vi "File Read Binary File.vi"(5 "count":i32=-1, 6 "字节顺序":T1(ring)=enum."little-endian", 8 "error in":errorcluster, 9 "access":enum16{"read/write", "read-only", "write-only"}(ring)=enum."read-only", 10 "operation":T2(ring), 11 "file path":path) -> (0 "error Output":errorcluster, 2 "Variant Output":variant, 3 "path":path)   [LabVIEW 2018]
doc: "从字节流二进制文件中读取数据数组。默认情况下，VI被配置为读取8字节Little Endian数据（双精度长整型DBL）。要修改从文件中读取采样数据的方式，可修改字节顺序和字节大小的值（通常大小为1、2、4或8）。如修改字节大小，也需修改数据类型常量的表示法，使其与字节大小相一致（1 = I8、2 = I16、4 = I32、8 = DBL）。用“写入二进制文件”VI创建文件。"
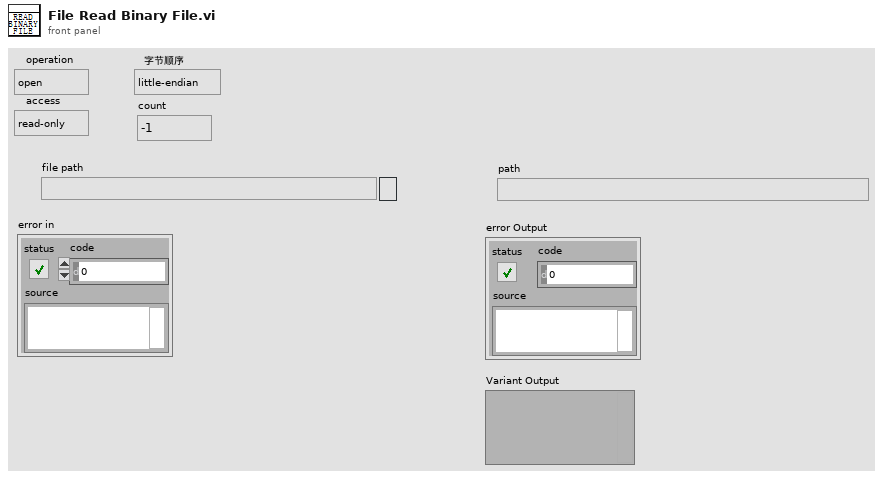
[diagram p1: front panel]
types:
  T1 = enum16{"big-endian, network order", "native, host order", "little-endian"}
  T2 = enum16{"open", "replace", "create", "open or create", "replace or create", "replace or create with confirmation"}
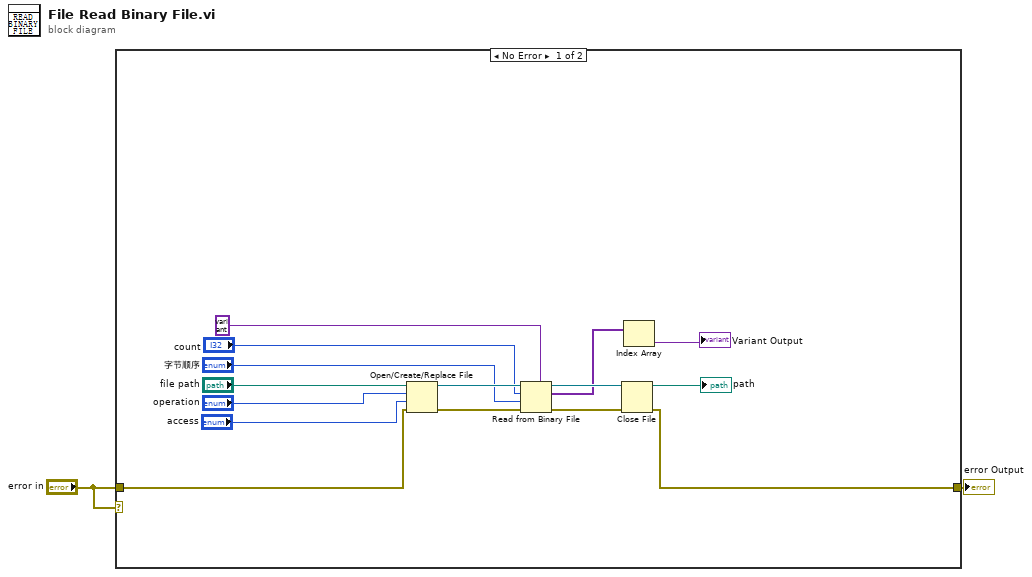
[diagram p0: block diagram]
diagram:
  n1 = case shown="No Error" "error in" {
    tunnel: "error in" -> [w7 w18]
    tunnel: [w3 w18] -> w1
    frame No Error {
      n2 = Open/Create/Replace File(file path (use dialog)="file path", error in=w7, operation (0:open)="operation", access (0:read/write)="access") -> (refnum out=w13:refnum<file>, error out=w14:errorcluster)  [unwired: 2 in, 1 out]
      n3 = Read from Binary File(5:variant, 8:w14, 9:"字节顺序", 10:"count", 11:w13) -> (0:w8:errorcluster, 2:w6:variant[], 3:w17:refnum<file>)  [unwired: 1 in, 1 out]
      n4 = Close File(refnum=w17, error in=w8) -> (path=→"path":path, error out=w3:errorcluster)
      n5 = Index Array(array=w6) -> (element=→"Variant Output":variant)  [unwired: 1 in]
    }
    frame Error {
    }
  }
  "error Output" <- w1
